vi "FCI_(Display presence absence).vi"(11 "Display Array":string[][](array[string])) -> (3 "Display Array":string[][](array[string]))   [LabVIEW 2015, in "ZenGage v3.0 UI.lvclass"]
uses:
  ZenGage v3.0 UI.lvclass
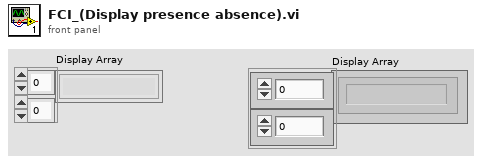
[diagram p1: front panel]
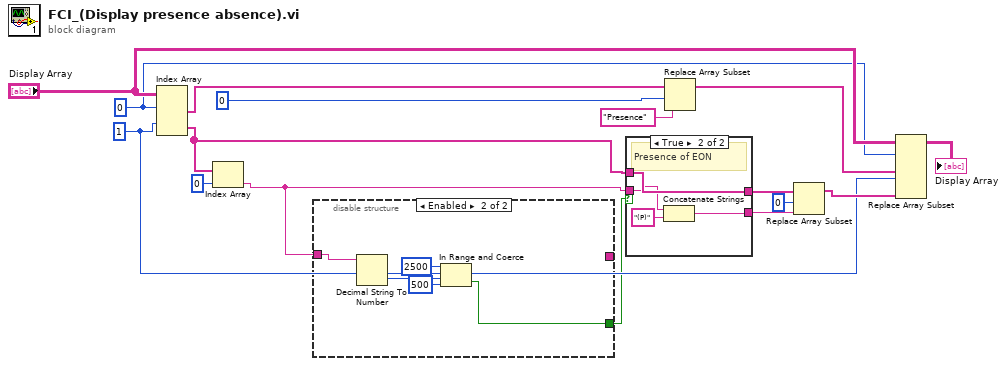
[diagram p0: block diagram]
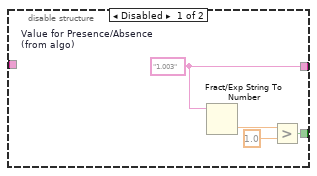
[diagram p2: hidden frame]
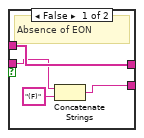
[diagram p3: hidden frame]
diagram:
  w3 = 1 ("index")
  w4 = 0 ("index")
  n1 = Index Array(array="Display Array", index (row) #1=w4, index (row) #2=w3) -> (element #1=w16:string[], element #2=w13:string[])  [unwired: 2 in]
  n2 = Index Array(array=w13, index=0) -> (element=w1:string)
  n3 = disable-structure shown="Enabled" {
    disable-tunnel: [w20 _] -> _
    disable-tunnel: [w17 w21] -> w2
    disable-tunnel: w1 -> [_ w25]
    frame Disabled {
      w20 = "1.003"  # Value for Presence/Absence (from algo)
      n4 = Fract/Exp String To Number(string=w20) -> (number=w19:dbl)  [unwired: 3 in, 1 out]
      n5 = Greater?(x=w19, y=1.0) -> (0:w17:bool)
    }
    frame Enabled {
      n6 = Decimal String To Number(string=w25) -> (number=w24:i32)  [unwired: 2 in, 1 out]
      n7 = In Range and Coerce(upper limit=2500, x=w24, lower limit=500) -> (In Range?=w21:bool)  [unwired: 1 out]
    }
  }
  n8 = case shown="True" w2 {
    tunnel: w13 -> [w29 w33]
    tunnel: [w29 w33] -> w12
    tunnel: [w27 w30] -> w11
    tunnel: w1 -> [w26 w32]
    frame False {
      # "Absence of EON"
      n9 = Concatenate Strings(w26, "(F)" ("string")) -> (w27:string)
    }
    frame True {
      # "Presence of EON"
      n10 = Concatenate Strings(w32, "(P)" ("string")) -> (w30:string)
    }
  }
  n11 = Replace Array Subset(array=w16, new element="Presence" ("new element/subarray"), index=0) -> (w7:string[])
  n12 = Replace Array Subset(array=w12, new element=w11, index=0) -> (w6:string[])
  n13 = Replace Array Subset(array="Display Array", new element #1=w7, index (row) #1=w4, new element #2=w6, index (row) #2=w3) -> (→"Display Array":string[][])  [unwired: 2 in]
